vi "CLD 2  Elapsed Time Express Caller Solution.vi"() -> ()   [LabVIEW 2020]
doc: "CLD 2 Exercise"
panel:
  out "Time Has Elapsed":bool
  out "Elapsed Time (s)":dbl format="%#.2g"
  out "error out":errorcluster
  in  "Time Target (s)":dbl=4.0
  in  "Auto Reset (F)":bool=TRUE
  in  "error in (no error)":errorcluster
  in  "Timer Mode":enum16{"Reset", "Read Status", "Set Auto Reset"}(ring)
  in  "stop":bool
  # "Caller for the FGV"
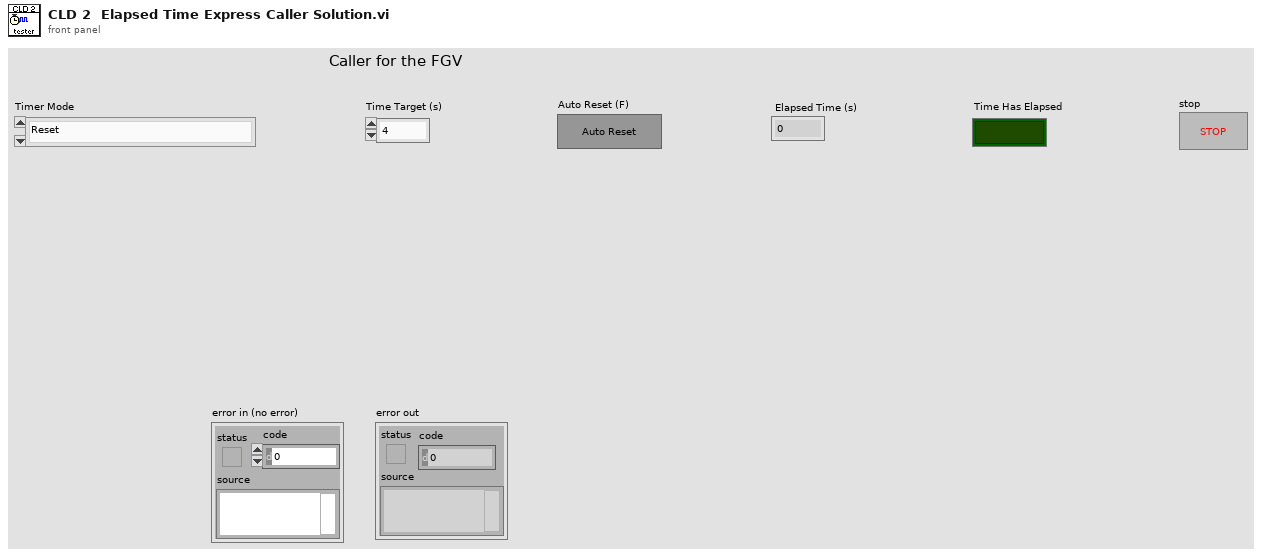
[diagram p1: front panel]
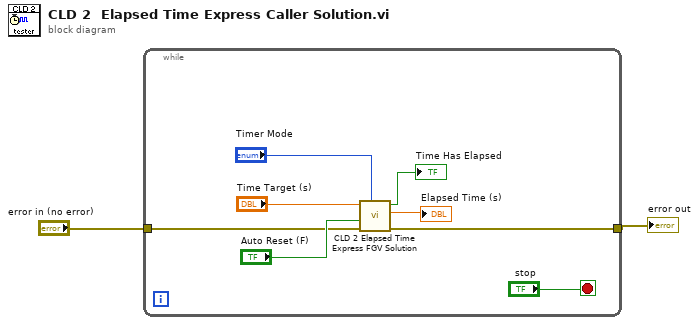
[diagram p0: block diagram]
diagram:
  n1 = while {
    tunnel: "error in (no error)" -> [w5]
    tunnel: [w4] -> w1
    stop <- "stop" stop-if-true
    n2 = call "CLD 2 Elapsed Time Express FGV Solution.vi"("Express Timer FGV Enum"="Timer Mode", "error in (no error)"=w5, "Auto Reset (F)"="Auto Reset (F)", "Time Target (s)"="Time Target (s)") -> ("error out"=w4:errorcluster, "Elapsed Time (s)"=→"Elapsed Time (s)":dbl, "Time Has Elapsed"=→"Time Has Elapsed":bool)  [unwired: 5 in]
  }
  "error out" <- w1
